vi "Generate-Screenshots-Top.vi"() -> ()   [LabVIEW 2017]
panel:
  out "Failed to Convert (File could be empty)":path[](array[path])
  out "Files to Convert":path[](array[path])
  in  "Source Directory":path=path "Z:/work/git/ScreenShotGen"
  # "Select Source Directory then run this vi.  \n* Generates a -Front.png and -Back.png screenshot for each vi.\n* Files that fail are simply skipped\n* Recursive"
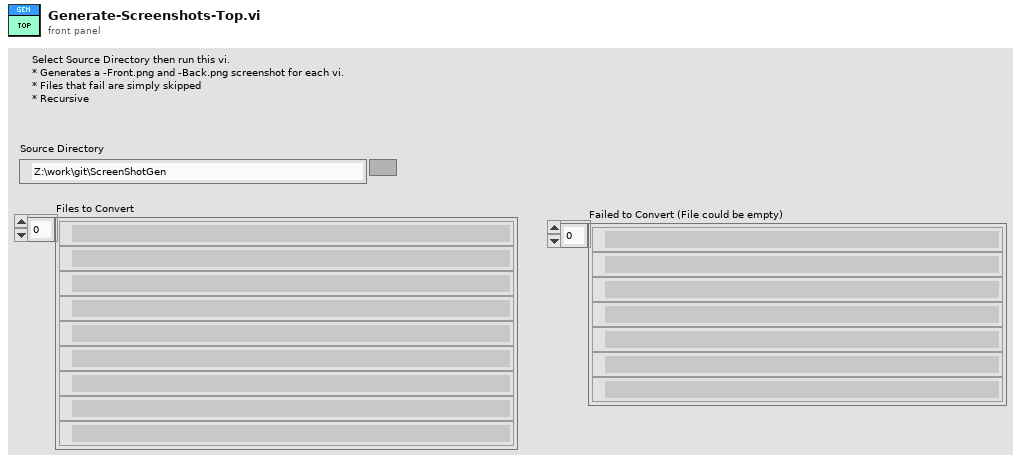
[diagram p1: front panel]
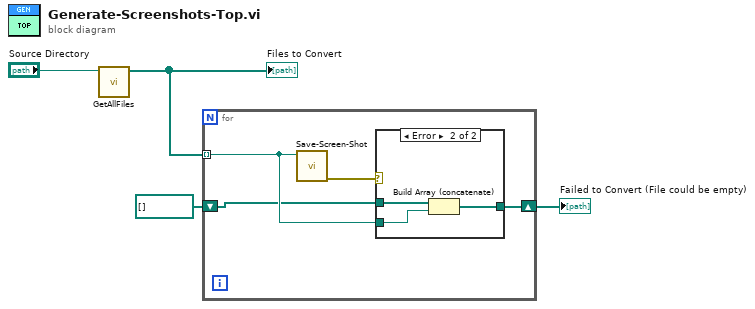
[diagram p0: block diagram]
diagram:
  n1 = call "GetAllFiles.vi"("Source Directory"="Source Directory") -> ("Files"=w3:path[])  [unwired: 9 in, 1 out]
  "Files to Convert" <- w3
  n2 = for {
    tunnel: w3 -> [w7] mode=indexing
    shift-right: [w6] -> w1
    shift-left: path[] [] -> [w5]
    n3 = call "Save-Screen-Shot.vi"("VI Path"=w7) -> ("error out"=w8:errorcluster)  [unwired: 10 in]
    n4 = case shown="Error" w8 {
      tunnel: w7 -> [_ w12]
      tunnel: [w9 w11] -> w6
      tunnel: w5 -> [w9 w10]
      frame No Error {
      }
      frame Error {
        n5 = Build Array (concatenate)(w10, w12) -> (w11:path[])
      }
    }
  }
  "Failed to Convert (File could be empty)" <- w1
